vi "ManagerEventExe.vi"(8 "error in (no error)":errorcluster, 10 "Event Registration Refnum In":refnum<event-registration>, 11 "Manager In":u64 caption="Device In") -> (0 "error out":errorcluster, 1 "phid":u64, 2 "Event Registration Refnum Out":refnum<event-registration>, 3 "Manager Out":u64 caption="Device Out", 4 "Timed Out?":bool, 5 "Event?":bool)   [LabVIEW 2012, in "Phidget Manager.lvlib"]
doc: "${AccelerationChange:Header}"
uses:
  <instrlib>/Phidgets/Phidget Manager/Phidget Manager.lvlib
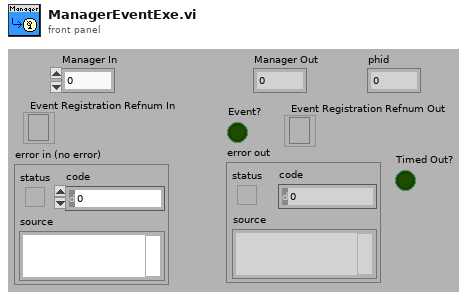
[diagram p1: front panel]
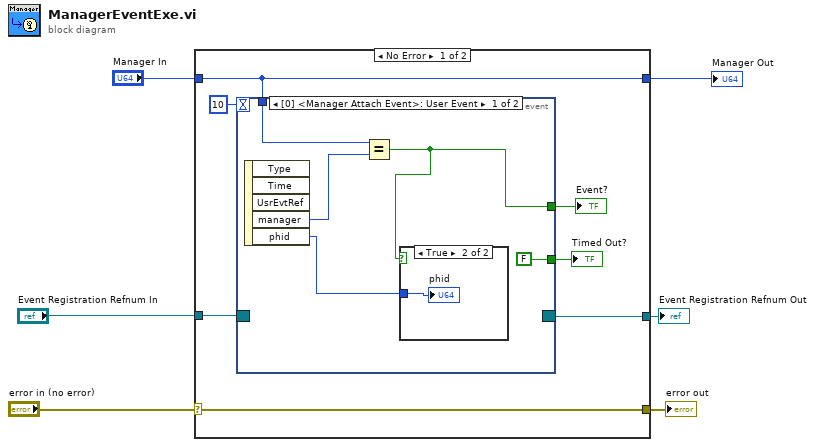
[diagram p0: block diagram]
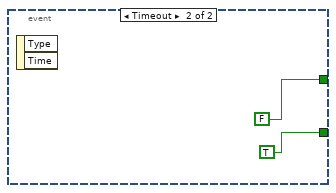
[diagram p3: hidden frame]
diagram:
  n1 = case shown="No Error" "error in (no error)" {
    selector: "error in (no error)" -> [w10 w24]
    tunnel: [w10 w24] -> w5
    tunnel: [w13 w23] -> w3
    tunnel: "Event Registration Refnum In" -> [w12 w23]
    tunnel: [w9 w22] -> w1
    tunnel: "Manager In" -> [w9 w22]
    frame No Error {
      n2 = event shown="[0] <Manager Attach Event>: User Event" {
        selector: w12 -> [_ _]
        dyn-events: [_ _] -> w13
        timeout: 10 -> [_ _]
        tunnel: [w15 FALSE] -> w11
        tunnel: w9 -> [w17 _]
        tunnel: [FALSE TRUE] -> w7
        event User Event {
          n3 = event-data() -> ("manager"=w16:u64, "phid"=w18:u64)  [unwired: 1 in, 3 out]
          n4 = Equal?(x=w17, y=w16) -> (x = y?=w15:bool)
          n5 = case shown="True" w15 {
            tunnel: w18 -> [_ w19]
            frame False {
            }
            frame True {
              "phid" <- w19
            }
          }
        }
        event Timeout {
          n6 = event-data() -> ()  [unwired: 1 in, 2 out]
        }
      }
      "Event?" <- w11
      "Timed Out?" <- w7
    }
    frame Error {
    }
  }
  "error out" <- w5
  "Event Registration Refnum Out" <- w3
  "Manager Out" <- w1
